vi "merFISH_create_tasks_list.vi"(2 "Probe List Refnum":refnum<vi>, 3 "error in":errorcluster, 4 "merFISH path":path=path "E:/", 5 "N ROIs":i32) -> (0 "Task list":T1[](array[typedef]), 1 "refnum log file":refnum<file>)   [LabVIEW 2015]
uses:
  CONTROLS/Q_main_element.ctl
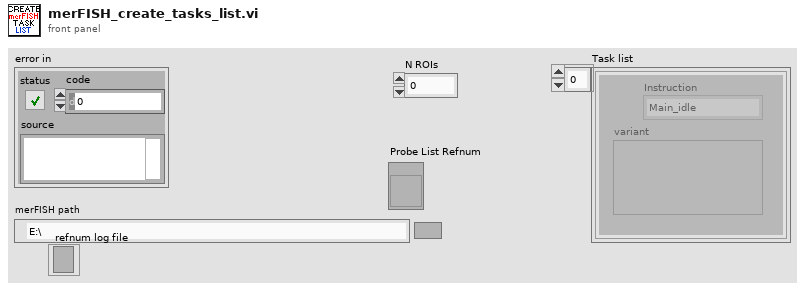
[diagram p1: front panel]
types:
  T1 = typedef "Q_main_element.ctl" = cluster{"variant":variant, "Instruction":enum16{"Main_idle", "Main_initialize", "Main_initialize_TDMS", "Main_initialize_Queue", "Main_error", "Main_DAQ_initialization_results", "Main_ASI_initialization_results", "Main_Piezo_initialization_results", "Main_Valve_initialization_results", "Main_Pump_initialization_results", "Main_CAMERA_initialization_results", "Main_DAQ_error", "Main_ASI_error", "Main_Piezo_error", "Main_CAMERA_error", "Main_Valve_error", "Main_Pump_error", "Main_start_acquiring", "Main_not_acquiring", "Main_acquiring", "Main_stop_acquiring", "Main_change_exposure", "Main_change_z_scan_parameters", "Main_define_ROI", "Main_read_kinetic_time", "Main_cooler", "Main_read_temperature", "Main_save_XY", "Main_load_XY", "Main_discard_XY", "Main_move_to_XY", "Main_measure_QPD", "Main_autofocus_calibration", "Main_save_PID", "Main_change_H_valve_position", "Main_two_way_valve", "Main_save_movie", "Main_init_single_scan", "Main_single_scan", "Main_stop_single_scan", "Main_merFISH_illumination_parameters", "Main_merFISH_buffer_probe_list", "Main_merFISH_injections_procedure", "Main_merFISH_save_setpoint", "Main_merFISH_init", "Main_merFISH_start_autofocus", "Main_merFISH_open_close_valve_merFISH", "Main_merFISH_open_close_valve_photobleaching", "Main_merFISH_hybridization", "Main_merFISH_move_to_ROI", "Main_merFISH_wait_stabilization", "Main_merFISH_scan", "Main_merFISH_photobleaching_injection", "Main_merFISH_photobleaching", "Main_merFISH_save", "Main_merFISH_send_email", "Main_merFISH_close", "Main_TL_define_parameters", "Main_TL_init", "Main_TL_start_autofocus", "Main_TL_move_to_ROI", "Main_TL_wait_for_stabilization", "Main_TL_scan", "Main_TL_wait_cycle_end", "Main_TL_close", "Main_STOP"}}
  T2 = enum16{"open", "replace", "create", "open or create", "replace or create", "replace or create with confirmation"}
  T3 = enum16{"Left Button", "Center Button", "Right Button", "Window Close"}
  T4 = cluster{"ROI #":i32, "Probe #":i32, "Folder# ":i32}
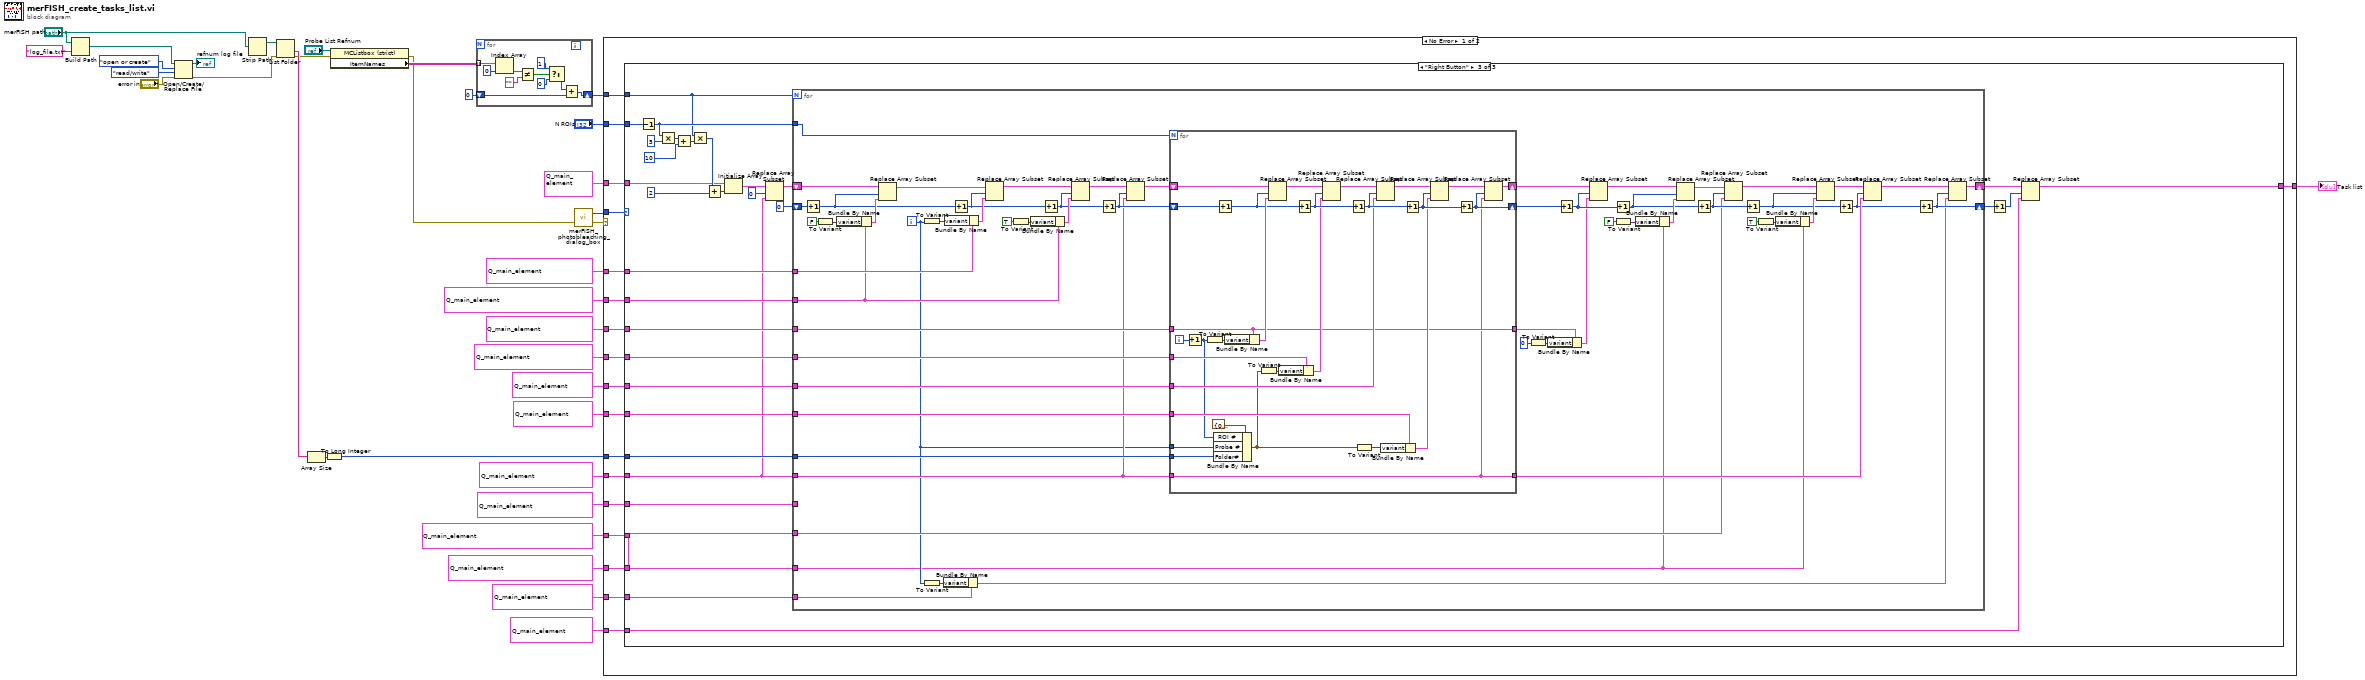
[diagram p0: block diagram]
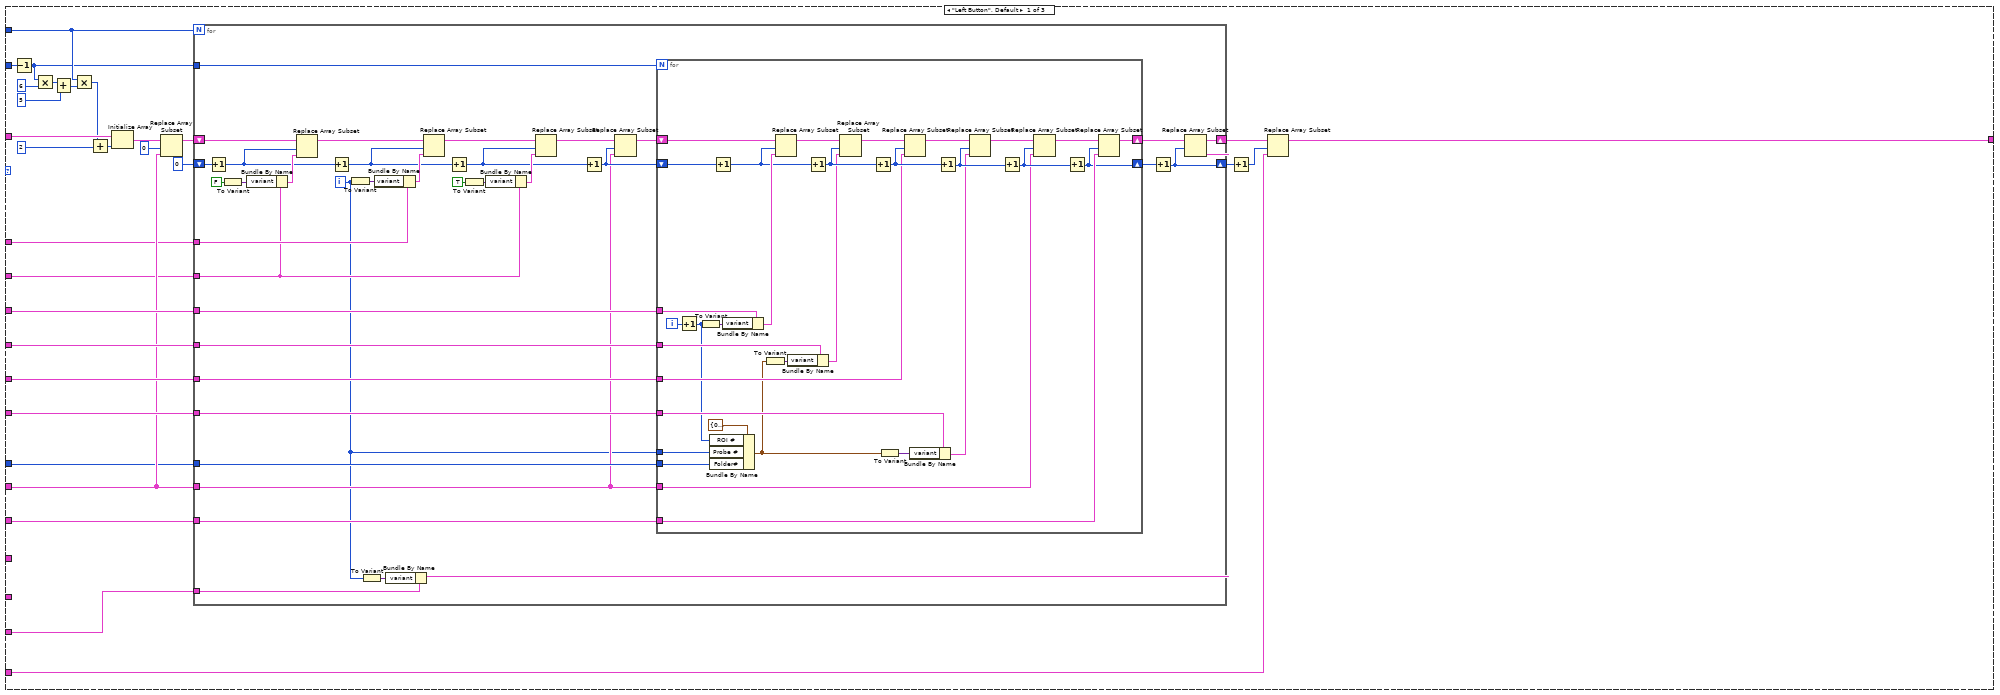
[diagram p2: hidden frame]
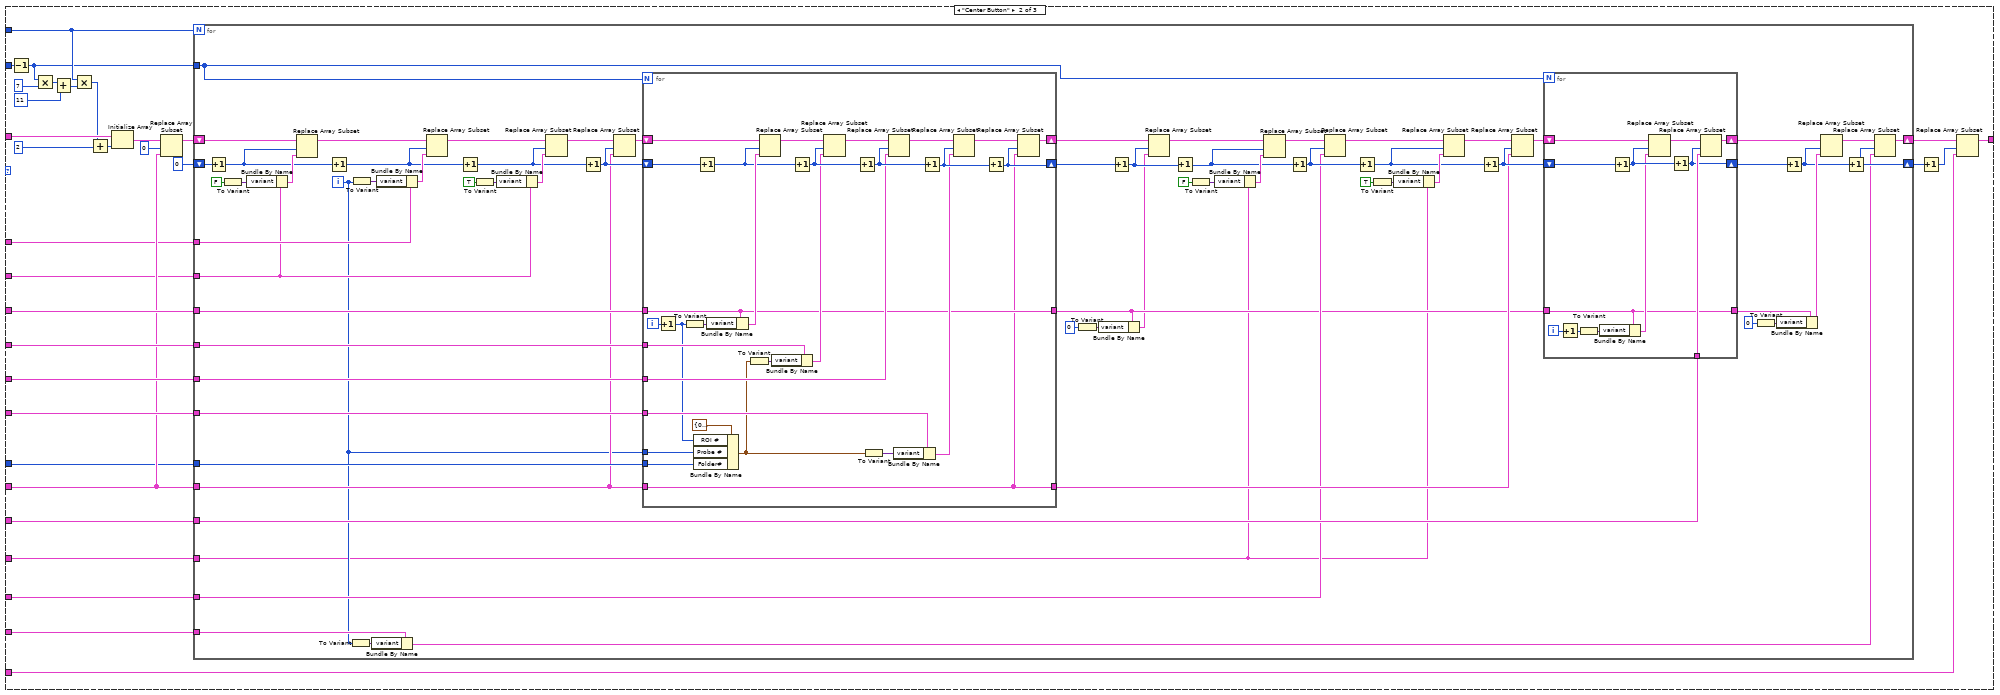
[diagram p3: hidden frame]
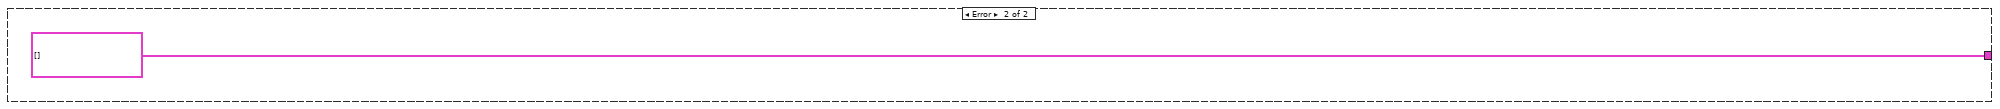
[diagram p4: hidden frame]
diagram:
  n1 = Build Path(base path="merFISH path", name or relative path="log_file.txt") -> (appended path=w13:path)
  n2 = Open/Create/Replace File(file path (use dialog)=w13, error in="error in", operation (0:open)=T2."open or create", access (0:read/write)=enum16{"read/write", "read-only", "write-only"}."read/write") -> (refnum out=→"refnum log file":refnum<file>, error out=w8:errorcluster)  [unwired: 2 in, 1 out]
  n3 = Strip Path(path="merFISH path") -> (stripped path=w7:path)  [unwired: 1 out]
  n4 = List Folder(path=w7, error in=w8) -> (folder names=w22:string[], error out=w20:errorcluster)  [unwired: 2 in, 2 out]
  n5 = Array Size(array=w22) -> (size(s)=w21:i32)
  n6 = To Long Integer(number=w21) -> (32bit integer=w19:i32)
  n7 = property class="MCListbox (strict)"(reference="Probe List Refnum", error in=w20) -> (error out=w1:errorcluster, "ItemNames"=w25:string[][])  [unwired: 1 out]
  n8 = for {
    tunnel: w25 -> [w45] mode=indexing
    shift-right: [w38] -> w23
    shift-left: 0 ("f") -> [w36]
    n9 = Index Array(array=w45, index=0) -> (element=w43:string)
    n10 = Not Equal?(x=w43, y="") -> (x != y?=w41:bool)
    n11 = Select(t=1, s=w41, f=0) -> (s? t:f=w37:i32)
    n12 = Add(x=w37, y=w36) -> (x+y=w38:i32)
  }
  n13 = call "merFISH_photobleaching_dialog_box.vi"("error in"=w1) -> ("error out"=w6:errorcluster, "Which Button?"=w5:T3)  [unwired: 1 in]
  n14 = case shown="No Error" w6 {
    tunnel: [w63 T1[] []] -> w2
    tunnel: T1 {"variant"=variant, "Instruction"=enum."Main_idle"} ("element") -> [w62 _]
    tunnel: T1 {"variant"=variant, "Instruction"=enum."Main_merFISH_move_to_ROI"} ("element") -> [w61 _]
    tunnel: T1 {"variant"=variant, "Instruction"=enum."Main_merFISH_wait_stabilization"} ("element") -> [w60 _]
    tunnel: T1 {"variant"=variant, "Instruction"=enum."Main_merFISH_scan"} ("element") -> [w59 _]
    tunnel: T1 {"variant"=variant, "Instruction"=enum."Main_merFISH_save"} ("element") -> [w58 _]
    tunnel: T1 {"variant"=variant, "Instruction"=enum."Main_merFISH_close"} ("element") -> [w57 _]
    tunnel: T1 {"variant"=variant, "Instruction"=enum."Main_merFISH_start_autofocus"} ("element") -> [w55 _]
    tunnel: T1 {"variant"=variant, "Instruction"=enum."Main_merFISH_photobleaching"} ("element") -> [w56 _]
    tunnel: T1 {"variant"=variant, "Instruction"=enum."Main_merFISH_hybridization"} ("element") -> [w54 _]
    tunnel: w23 -> [w53 _]
    tunnel: w19 -> [w52 _]
    tunnel: T1 {"variant"=variant, "Instruction"=enum."Main_merFISH_open_close_valve_merFISH"} ("element") -> [w51 _]
    tunnel: w5 -> [w50 _]
    tunnel: "N ROIs" -> [w49 _]
    tunnel: T1 {"variant"=variant, "Instruction"=enum."Main_merFISH_photobleaching_injection"} ("element") -> [w48 _]
    tunnel: T1 {"variant"=variant, "Instruction"=enum."Main_merFISH_send_email"} ("element") -> [w47 _]
    tunnel: T1 {"variant"=variant, "Instruction"=enum."Main_merFISH_open_close_valve_photobleaching"} ("element") -> [w46 _]
    frame No Error {
      n15 = case shown="\"Right Button\"" w50 {
        tunnel: [w89 w189 w304] -> w63
        tunnel: w62 -> [w87 w187 w314]
        tunnel: w61 -> [w86 w186 w312]
        tunnel: w60 -> [w85 w185 w311]
        tunnel: w59 -> [w84 w184 w310]
        tunnel: w58 -> [w83 w183 w309]
        tunnel: w57 -> [w82 w182 w305]
        tunnel: w56 -> [w79 w166 w306]
        tunnel: w55 -> [w78 w179 w307]
        tunnel: w54 -> [w76 w177 w315]
        tunnel: w53 -> [w71 w172 w317]
        tunnel: w52 -> [w70 w171 w308]
        tunnel: w51 -> [w69 w170 w313]
        tunnel: w49 -> [w66 w167 w316]
        tunnel: w48 -> [_ w165 w302]
        tunnel: w47 -> [w64 w163 w303]
        tunnel: w46 -> [_ w162 _]
        frame "Left Button", Default {
          n16 = Decrement(x=w66) -> (x-1=w65:i32)
          n17 = Multiply(x=w65, y=6) -> (x*y=w68:i32)
          n18 = Add(x=w68, y=5) -> (x+y=w75:i32)
          n19 = Multiply(x=w71, y=w75) -> (x*y=w74:i32)
          n20 = Add(x=w74, y=2) -> (x+y=w73:i32)
          n21 = Initialize Array(w87, w73) -> (w81:T1[])
          n22 = Replace Array Subset(array=w81, new element=w78, index=0) -> (w77:T1[])
          n23 = for {
            N: w71 -> [_]
            tunnel: w86 -> [w129]
            tunnel: w85 -> [w128]
            tunnel: w84 -> [w127]
            tunnel: w83 -> [w126]
            tunnel: w79 -> [w125]
            tunnel: w78 -> [w104]
            shift-right: [w98] -> w91
            shift-left: 0 -> [w118]
            shift-right: [w99] -> w88
            shift-left: w77 -> [w119]
            tunnel: w65 -> [w124]
            tunnel: w76 -> [w110]
            tunnel: w70 -> [w121]
            tunnel: w69 -> [w109]
            tunnel: w64 -> [w95]
            i -> [w96]
            n24 = Increment(x=w118) -> (x+1=w103:i32)
            n25 = To Variant(anything=FALSE) -> (Variant=w120:variant)
            n26 = Bundle By Name(cluster=w109, "variant"=w120) -> (w116:T1)
            n27 = Replace Array Subset(array=w119, new element=w116, index=w103) -> (w102:T1[])
            n28 = Increment(x=w103) -> (x+1=w111:i32)
            n29 = To Variant(anything=w96) -> (Variant=w123:variant)
            n30 = To Variant(anything=w96) -> (Variant=w97:variant)
            n31 = Bundle By Name(cluster=w110, "variant"=w123) -> (w122:T1)
            n32 = Bundle By Name(cluster=w95, "variant"=w97) -> (w94:T1)
            n33 = Replace Array Subset(array=w102, new element=w122, index=w111) -> (w112:T1[])
            n34 = Increment(x=w111) -> (x+1=w106:i32)
            n35 = To Variant(anything=TRUE) -> (Variant=w113:variant)
            n36 = Bundle By Name(cluster=w109, "variant"=w113) -> (w115:T1)
            n37 = Replace Array Subset(array=w112, new element=w115, index=w106) -> (w107:T1[])
            n38 = Increment(x=w106) -> (x+1=w105:i32)
            n39 = Replace Array Subset(array=w107, new element=w104, index=w105) -> (w108:T1[])
            n40 = for {
              N: w124 -> [_]
              shift-right: [w147] -> w101
              shift-left: w108 -> [w154]
              tunnel: w129 -> [w151]
              tunnel: w128 -> [w133]
              tunnel: w127 -> [w148]
              tunnel: w126 -> [w150]
              tunnel: w125 -> [w144]
              tunnel: w104 -> [w140]
              shift-right: [w143] -> w100
              shift-left: w105 -> [w139]
              tunnel: w96 -> [w136]
              tunnel: w121 -> [w135]
              i -> [w137]
              n41 = Increment(x=w137) -> (x+1=w130:i32)
              n42 = To Variant(anything=w130) -> (Variant=w161:variant)
              n43 = Bundle By Name(cluster=T4 {"ROI #"=0, "Probe #"=0, "Folder# "=0}, "ROI #"=w130, "Probe #"=w136, "Folder#"=w135) -> (w131:T4)
              n44 = Increment(x=w139) -> (x+1=w142:i32)
              n45 = Bundle By Name(cluster=w151, "variant"=w161) -> (w149:T1)
              n46 = To Variant(anything=w131) -> (Variant=w134:variant)
              n47 = Replace Array Subset(array=w154, new element=w149, index=w142) -> (w153:T1[])
              n48 = Bundle By Name(cluster=w133, "variant"=w134) -> (w132:T1)
              n49 = Increment(x=w142) -> (x+1=w152:i32)
              n50 = Replace Array Subset(array=w153, new element=w132, index=w152) -> (w160:T1[])
              n51 = Increment(x=w152) -> (x+1=w158:i32)
              n52 = To Variant(anything=w131) -> (Variant=w155:variant)
              n53 = Replace Array Subset(array=w160, new element=w148, index=w158) -> (w159:T1[])
              n54 = Bundle By Name(cluster=w150, "variant"=w155) -> (w141:T1)
              n55 = Increment(x=w158) -> (x+1=w156:i32)
              n56 = Replace Array Subset(array=w159, new element=w141, index=w156) -> (w157:T1[])
              n57 = Increment(x=w156) -> (x+1=w145:i32)
              n58 = Replace Array Subset(array=w157, new element=w140, index=w145) -> (w146:T1[])
              n59 = Increment(x=w145) -> (x+1=w143:i32)
              n60 = Replace Array Subset(array=w146, new element=w144, index=w143) -> (w147:T1[])
            }
            n61 = Increment(x=w100) -> (x+1=w98:i32)
            n62 = Replace Array Subset(array=w101, new element=w94, index=w98) -> (w99:T1[])
          }
          n63 = Increment(x=w91) -> (x+1=w90:i32)
          n64 = Replace Array Subset(array=w88, new element=w82, index=w90) -> (w89:T1[])
        }
        frame "Center Button" {
          n65 = Decrement(x=w167) -> (x-1=w164:i32)
          n66 = Multiply(x=w164, y=7) -> (x*y=w169:i32)
          n67 = Add(x=w169, y=11) -> (x+y=w176:i32)
          n68 = Multiply(x=w172, y=w176) -> (x*y=w175:i32)
          n69 = Add(x=w175, y=2) -> (x+y=w174:i32)
          n70 = Initialize Array(w187, w174) -> (w181:T1[])
          n71 = Replace Array Subset(array=w181, new element=w179, index=0) -> (w178:T1[])
          n72 = for {
            N: w172 -> [_]
            tunnel: w186 -> [w260]
            tunnel: w185 -> [w259]
            tunnel: w184 -> [w258]
            tunnel: w183 -> [w257]
            tunnel: w179 -> [w238]
            shift-right: [w199] -> w191
            shift-left: 0 -> [w251]
            shift-right: [w201] -> w188
            shift-left: w178 -> [w252]
            tunnel: w164 -> [w236]
            tunnel: w177 -> [w243]
            tunnel: w171 -> [w254]
            tunnel: w170 -> [w223]
            tunnel: w166 -> [w237]
            tunnel: w165 -> [w221]
            tunnel: w163 -> [w197]
            tunnel: w162 -> [w194]
            i -> [w195]
            n73 = Increment(x=w251) -> (x+1=w206:i32)
            n74 = To Variant(anything=FALSE) -> (Variant=w253:variant)
            n75 = Bundle By Name(cluster=w223, "variant"=w253) -> (w249:T1)
            n76 = Replace Array Subset(array=w252, new element=w249, index=w206) -> (w205:T1[])
            n77 = Increment(x=w206) -> (x+1=w244:i32)
            n78 = To Variant(anything=w195) -> (Variant=w198:variant)
            n79 = To Variant(anything=w195) -> (Variant=w256:variant)
            n80 = Bundle By Name(cluster=w197, "variant"=w198) -> (w196:T1)
            n81 = Bundle By Name(cluster=w243, "variant"=w256) -> (w255:T1)
            n82 = Replace Array Subset(array=w205, new element=w255, index=w244) -> (w245:T1[])
            n83 = Increment(x=w244) -> (x+1=w240:i32)
            n84 = To Variant(anything=TRUE) -> (Variant=w246:variant)
            n85 = Bundle By Name(cluster=w223, "variant"=w246) -> (w248:T1)
            n86 = Replace Array Subset(array=w245, new element=w248, index=w240) -> (w241:T1[])
            n87 = Increment(x=w240) -> (x+1=w239:i32)
            n88 = Replace Array Subset(array=w241, new element=w238, index=w239) -> (w242:T1[])
            n89 = for {
              N: w236 -> [_]
              shift-right: [w276] -> w220
              shift-left: w242 -> [w294]
              tunnel: w260 -> [w275]
              tunnel: w259 -> [w280]
              tunnel: w258 -> [w289]
              tunnel: w257 -> [w291]
              tunnel: w238 -> [w274]
              shift-right: [w277] -> w219
              shift-left: w239 -> [w286]
              tunnel: w195 -> [w283]
              tunnel: w254 -> [w282]
              tunnel: [w275] -> w215
              tunnel: [w274] -> w222
              i -> [w284]
              n90 = Increment(x=w284) -> (x+1=w273:i32)
              n91 = To Variant(anything=w273) -> (Variant=w301:variant)
              n92 = Bundle By Name(cluster=T4 {"ROI #"=0, "Probe #"=0, "Folder# "=0}, "ROI #"=w273, "Probe #"=w283, "Folder#"=w282) -> (w278:T4)
              n93 = Increment(x=w286) -> (x+1=w288:i32)
              n94 = Bundle By Name(cluster=w275, "variant"=w301) -> (w290:T1)
              n95 = To Variant(anything=w278) -> (Variant=w281:variant)
              n96 = Replace Array Subset(array=w294, new element=w290, index=w288) -> (w293:T1[])
              n97 = Bundle By Name(cluster=w280, "variant"=w281) -> (w279:T1)
              n98 = Increment(x=w288) -> (x+1=w292:i32)
              n99 = Replace Array Subset(array=w293, new element=w279, index=w292) -> (w300:T1[])
              n100 = Increment(x=w292) -> (x+1=w298:i32)
              n101 = To Variant(anything=w278) -> (Variant=w295:variant)
              n102 = Replace Array Subset(array=w300, new element=w289, index=w298) -> (w299:T1[])
              n103 = Bundle By Name(cluster=w291, "variant"=w295) -> (w287:T1)
              n104 = Increment(x=w298) -> (x+1=w296:i32)
              n105 = Replace Array Subset(array=w299, new element=w287, index=w296) -> (w297:T1[])
              n106 = Increment(x=w296) -> (x+1=w277:i32)
              n107 = Replace Array Subset(array=w297, new element=w274, index=w277) -> (w276:T1[])
            }
            n108 = To Variant(anything=0) -> (Variant=w216:variant)
            n109 = Bundle By Name(cluster=w215, "variant"=w216) -> (w213:T1)
            n110 = Increment(x=w219) -> (x+1=w218:i32)
            n111 = Replace Array Subset(array=w220, new element=w213, index=w218) -> (w217:T1[])
            n112 = Increment(x=w218) -> (x+1=w204:i32)
            n113 = To Variant(anything=FALSE) -> (Variant=w235:variant)
            n114 = Bundle By Name(cluster=w194, "variant"=w235) -> (w233:T1)
            n115 = Replace Array Subset(array=w217, new element=w233, index=w204) -> (w203:T1[])
            n116 = Increment(x=w204) -> (x+1=w228:i32)
            n117 = Replace Array Subset(array=w203, new element=w221, index=w228) -> (w229:T1[])
            n118 = Increment(x=w228) -> (x+1=w226:i32)
            n119 = To Variant(anything=TRUE) -> (Variant=w230:variant)
            n120 = Bundle By Name(cluster=w194, "variant"=w230) -> (w232:T1)
            n121 = Replace Array Subset(array=w229, new element=w232, index=w226) -> (w227:T1[])
            n122 = Increment(x=w226) -> (x+1=w224:i32)
            n123 = Replace Array Subset(array=w227, new element=w222, index=w224) -> (w225:T1[])
            n124 = for {
              N: w236 -> [_]
              shift-right: [w270] -> w212
              shift-left: w225 -> [w272]
              shift-right: [w266] -> w211
              shift-left: w224 -> [w271]
              tunnel: w215 -> [w262]
              tunnel: w237 -> [w267]
              tunnel: [w262] -> w207
              i -> [w263]
              n125 = Increment(x=w263) -> (x+1=w261:i32)
              n126 = To Variant(anything=w261) -> (Variant=w265:variant)
              n127 = Bundle By Name(cluster=w262, "variant"=w265) -> (w264:T1)
              n128 = Increment(x=w271) -> (x+1=w268:i32)
              n129 = Replace Array Subset(array=w272, new element=w264, index=w268) -> (w269:T1[])
              n130 = Increment(x=w268) -> (x+1=w266:i32)
              n131 = Replace Array Subset(array=w269, new element=w267, index=w266) -> (w270:T1[])
            }
            n132 = To Variant(anything=0) -> (Variant=w209:variant)
            n133 = Bundle By Name(cluster=w207, "variant"=w209) -> (w208:T1)
            n134 = Increment(x=w211) -> (x+1=w200:i32)
            n135 = Replace Array Subset(array=w212, new element=w208, index=w200) -> (w202:T1[])
            n136 = Increment(x=w200) -> (x+1=w199:i32)
            n137 = Replace Array Subset(array=w202, new element=w196, index=w199) -> (w201:T1[])
          }
          n138 = Increment(x=w191) -> (x+1=w190:i32)
          n139 = Replace Array Subset(array=w188, new element=w182, index=w190) -> (w189:T1[])
        }
        frame "Right Button" {
          n140 = Decrement(x=w316) -> (x-1=w318:i32)
          n141 = Multiply(x=w318, y=5) -> (x*y=w320:i32)
          n142 = Add(x=w320, y=10) -> (x+y=w324:i32)
          n143 = Multiply(x=w317, y=w324) -> (x*y=w323:i32)
          n144 = Add(x=w323, y=2) -> (x+y=w322:i32)
          n145 = Initialize Array(w314, w322) -> (w327:T1[])
          n146 = Replace Array Subset(array=w327, new element=w307, index=0) -> (w325:T1[])
          n147 = for {
            N: w317 -> [_]
            tunnel: w312 -> [w390]
            tunnel: w311 -> [w389]
            tunnel: w310 -> [w388]
            tunnel: w309 -> [w387]
            tunnel: w307 -> [w368]
            shift-right: [w338] -> w330
            shift-left: 0 -> [w381]
            shift-right: [w341] -> w328
            shift-left: w325 -> [w382]
            tunnel: w318 -> [w367]
            tunnel: w315 -> [w373]
            tunnel: w308 -> [w384]
            tunnel: w313 -> [w356]
            tunnel: w306 -> [_]
            tunnel: w302 -> [w354]
            tunnel: w303 -> [w335]
            tunnel: w302 -> [w333]
            i -> [w334]
            n148 = Increment(x=w381) -> (x+1=w344:i32)
            n149 = To Variant(anything=FALSE) -> (Variant=w383:variant)
            n150 = Bundle By Name(cluster=w356, "variant"=w383) -> (w379:T1)
            n151 = Replace Array Subset(array=w382, new element=w379, index=w344) -> (w345:T1[])
            n152 = To Variant(anything=w334) -> (Variant=w386:variant)
            n153 = To Variant(anything=w334) -> (Variant=w337:variant)
            n154 = Bundle By Name(cluster=w335, "variant"=w337) -> (w336:T1)
            n155 = Bundle By Name(cluster=w373, "variant"=w386) -> (w385:T1)
            n156 = Increment(x=w344) -> (x+1=w374:i32)
            n157 = Replace Array Subset(array=w345, new element=w385, index=w374) -> (w375:T1[])
            n158 = To Variant(anything=TRUE) -> (Variant=w376:variant)
            n159 = Bundle By Name(cluster=w356, "variant"=w376) -> (w378:T1)
            n160 = Increment(x=w374) -> (x+1=w370:i32)
            n161 = Replace Array Subset(array=w375, new element=w378, index=w370) -> (w371:T1[])
            n162 = Increment(x=w370) -> (x+1=w369:i32)
            n163 = Replace Array Subset(array=w371, new element=w368, index=w369) -> (w372:T1[])
            n164 = for {
              N: w367 -> [_]
              shift-right: [w394] -> w353
              shift-left: w372 -> [w412]
              tunnel: w390 -> [w393]
              tunnel: w389 -> [w398]
              tunnel: w388 -> [w407]
              tunnel: w387 -> [w409]
              tunnel: w368 -> [w392]
              shift-right: [w395] -> w352
              shift-left: w369 -> [w404]
              tunnel: w334 -> [w401]
              tunnel: w384 -> [w400]
              tunnel: [w393] -> w348
              tunnel: [w392] -> w355
              i -> [w402]
              n165 = Increment(x=w402) -> (x+1=w391:i32)
              n166 = To Variant(anything=w391) -> (Variant=w419:variant)
              n167 = Bundle By Name(cluster=T4 {"ROI #"=0, "Probe #"=0, "Folder# "=0}, "ROI #"=w391, "Probe #"=w401, "Folder#"=w400) -> (w396:T4)
              n168 = Increment(x=w404) -> (x+1=w406:i32)
              n169 = Bundle By Name(cluster=w393, "variant"=w419) -> (w408:T1)
              n170 = To Variant(anything=w396) -> (Variant=w399:variant)
              n171 = Replace Array Subset(array=w412, new element=w408, index=w406) -> (w411:T1[])
              n172 = Bundle By Name(cluster=w398, "variant"=w399) -> (w397:T1)
              n173 = Increment(x=w406) -> (x+1=w410:i32)
              n174 = Replace Array Subset(array=w411, new element=w397, index=w410) -> (w418:T1[])
              n175 = Increment(x=w410) -> (x+1=w416:i32)
              n176 = To Variant(anything=w396) -> (Variant=w413:variant)
              n177 = Replace Array Subset(array=w418, new element=w407, index=w416) -> (w417:T1[])
              n178 = Bundle By Name(cluster=w409, "variant"=w413) -> (w405:T1)
              n179 = Increment(x=w416) -> (x+1=w414:i32)
              n180 = Replace Array Subset(array=w417, new element=w405, index=w414) -> (w415:T1[])
              n181 = Increment(x=w414) -> (x+1=w395:i32)
              n182 = Replace Array Subset(array=w415, new element=w392, index=w395) -> (w394:T1[])
            }
            n183 = To Variant(anything=0) -> (Variant=w349:variant)
            n184 = Bundle By Name(cluster=w348, "variant"=w349) -> (w346:T1)
            n185 = Increment(x=w352) -> (x+1=w351:i32)
            n186 = Replace Array Subset(array=w353, new element=w346, index=w351) -> (w350:T1[])
            n187 = Increment(x=w351) -> (x+1=w343:i32)
            n188 = To Variant(anything=FALSE) -> (Variant=w366:variant)
            n189 = Bundle By Name(cluster=w333, "variant"=w366) -> (w364:T1)
            n190 = Replace Array Subset(array=w350, new element=w364, index=w343) -> (w342:T1[])
            n191 = Increment(x=w343) -> (x+1=w359:i32)
            n192 = Replace Array Subset(array=w342, new element=w354, index=w359) -> (w360:T1[])
            n193 = Increment(x=w359) -> (x+1=w357:i32)
            n194 = To Variant(anything=TRUE) -> (Variant=w361:variant)
            n195 = Bundle By Name(cluster=w333, "variant"=w361) -> (w363:T1)
            n196 = Replace Array Subset(array=w360, new element=w363, index=w357) -> (w358:T1[])
            n197 = Increment(x=w357) -> (x+1=w339:i32)
            n198 = Replace Array Subset(array=w358, new element=w355, index=w339) -> (w340:T1[])
            n199 = Increment(x=w339) -> (x+1=w338:i32)
            n200 = Replace Array Subset(array=w340, new element=w336, index=w338) -> (w341:T1[])
          }
          n201 = Increment(x=w330) -> (x+1=w329:i32)
          n202 = Replace Array Subset(array=w328, new element=w305, index=w329) -> (w304:T1[])
        }
      }
    }
    frame Error {
    }
  }
  "Task list" <- w2
